vi "finalise_image.vi"(8 "error in (no error)":errorcluster, 9 "end of sweep?":bool, 11 "ImageAssemblerMG090623Binning in":refnum<class "ImageAssemblerMG090623Binning.lvclass">) -> (0 "error out":errorcluster, 3 "ImageAssemblerMG090623Binning out":refnum<class "ImageAssemblerMG090623Binning.lvclass">)   [LabVIEW 2010, in "ImageAssemblerMG090623Binning.lvclass"]
doc: "Finalises the image and sends it to registered observers. If the sweep is finished, a sweep terminator (empty Image array) is additionally send to observers."
uses:
  ImageAssemblerMG090623Binning.lvclass
  ImageAssemblerMG090623Binning.lvclass/ImageAssemblerMG090623Binning.ctl
  common/classes/Image/Image/Image.lvclass
  ImagingMode/GenericImagingMode/GenericImagingMode/GenericImagingMode.lvclass
  common/classes/GenericComponent/GenericComponent/class_data.vi
  common/classes/GenericComponent/GenericComponent/GenericComponent.lvclass
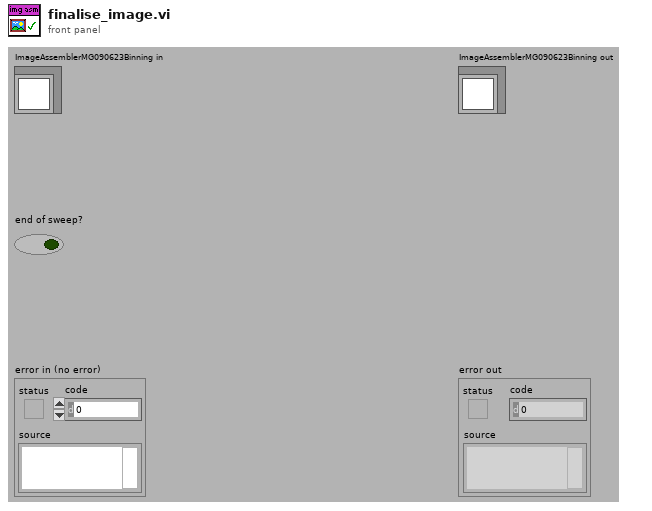
[diagram p1: front panel]
types:
  T1 = typedef "IMAQ Image.ctl" = refnum<image>
  T2 = typedef "GenericToplevelComponent.lvclass/common_trigger_enum.ctl" = enum16{"NULL", "initialise", "terminate", "fetch command", "fetch data", "attach observer", "register as observer", "detach observer", "acknowledge", "start", "stop", "sweep started", "sweep finished", "experiment started", "experiment stopped"}
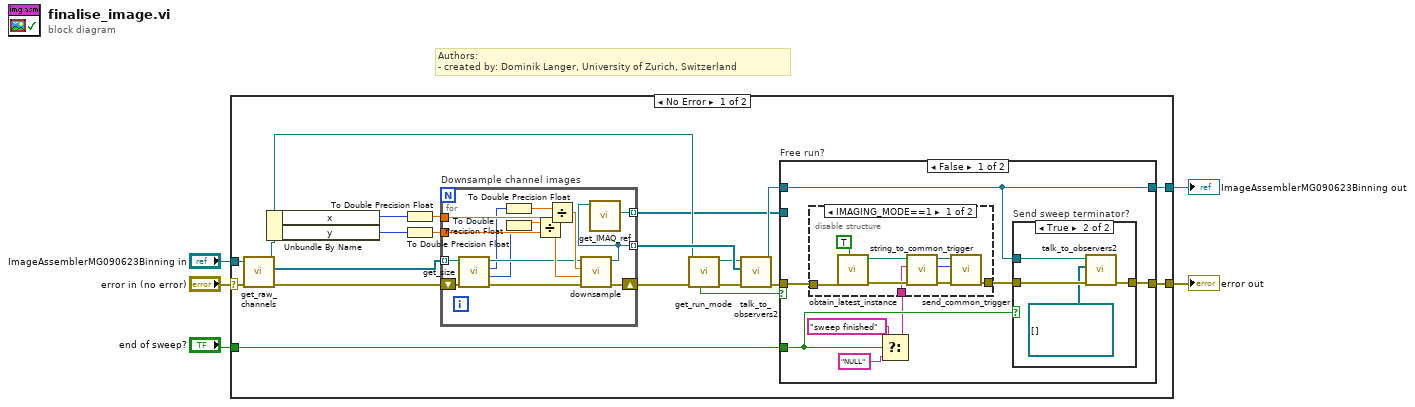
[diagram p0: block diagram]
diagram:
  # "Authors: \n- created by: Dominik Langer, University of Zurich, Switzerland"
  n1 = case shown="No Error" "error in (no error)" {
    selector: "error in (no error)" -> [w15 w67]
    tunnel: [w19 w67] -> w4
    tunnel: [w17 w66] -> w2
    tunnel: "ImageAssemblerMG090623Binning in" -> [w13 w66]
    tunnel: "end of sweep?" -> [w21 _]
    frame No Error {
      n2 = call-dynamic "get_raw_channels.vi"("error in (no error)"=w15, "DL090211ImageAssemblerScaffold.lvclass in"=w13) -> ("error out"=w14:errorcluster, "raw channels"=w11:refnum<class "Image.lvclass">[], "DL090211ImageAssemblerScaffold.lvclass out"=w12:refnum<class "ImageAssemblerMG090623Binning.lvclass">)  [unwired: 7 out]
      n3 = Unbundle By Name(w12) -> ("x"=w24:i32, "y"=w25:i32)
      n4 = To Double Precision Float(number=w24) -> (double precision float=w8:dbl)
      n5 = To Double Precision Float(number=w25) -> (double precision float=w7:dbl)
      n6 = for "Downsample channel images" {
        tunnel: w8 -> [w37]
        tunnel: w7 -> [w36]
        tunnel: w11 -> [w34] mode=indexing
        shift-right: [w28] -> w23
        shift-left: w14 -> [w35]
        tunnel: [w27] -> w16 mode=indexing
        tunnel: [w26] -> w6 mode=indexing
        n7 = call-dynamic "get_size.vi"("error in (no error)"=w35, "Image in"=w34) -> ("error out"=w40:errorcluster, "y resolution"=w31:i32, "x resolution"=w32:i32, "Image out"=w33:refnum<class "Image.lvclass">)  [unwired: 6 out]
        n8 = To Double Precision Float(number=w32) -> (double precision float=w29:dbl)
        n9 = To Double Precision Float(number=w31) -> (double precision float=w30:dbl)
        n10 = Divide(x=w30, y=w36) -> (x/y=w38:dbl)
        n11 = Divide(x=w29, y=w37) -> (x/y=w39:dbl)
        n12 = call-dynamic "downsample.vi"("error in (no error)"=w40, "y factor"=w38, "x factor"=w39, "Image in"=w33) -> ("error out"=w28:errorcluster, "Image out"=w27:refnum<class "Image.lvclass">)  [unwired: 6 out]
        n13 = call-dynamic "get_IMAQ_ref.vi"("Image.lvclass in"=w27) -> ("Image"=w26:T1)  [unwired: 6 in, 4 out]
      }
      n14 = call "get_run_mode.vi"("error in (no error)"=w23, "GenericPlugin in"=w12) -> ("error out"=w10:errorcluster, "GenericPlugin out"=w9:refnum<class "ImageAssemblerMG090623Binning.lvclass">, "is free run?"=w22:bool)  [unwired: 5 in, 2 out]
      n15 = call-dynamic "talk_to_observers2.vi"("error in (no error)"=w10, "image (channels)"=w16, "GenericToplevelComponent in"=w9) -> ("error out"=w20:errorcluster, "GenericToplevelComponent out"=w18:refnum<class "ImageAssemblerMG090623Binning.lvclass">)  [unwired: 7 in]
      n16 = case "Free run?" shown="False" w22 {
        tunnel: w20 -> [w48 w65]
        tunnel: [w46 w65] -> w19
        tunnel: w21 -> [w44 _]
        tunnel: w18 -> [w45 w64]
        tunnel: [w45 w64] -> w17
        tunnel: w6 -> [_ _]
        frame False {
          n17 = Select(t="sweep finished" ("message"), s=w44, f="NULL" ("message")) -> (s? t:f=w43:string)
          n18 = disable-structure shown="IMAGING_MODE==1" {
            disable-tunnel: w48 -> [w61 w63]
            disable-tunnel: [w60 w63] -> w47
            disable-tunnel: w43 -> [w54 _]
            frame condition #0 (active) {
              n19 = call "obtain_latest_instance.vi"("quick, but maybe outdated?"=TRUE, "error in (no error)"=w61) -> ("error out"=w59:errorcluster, "GenericScanMode out"=w57:refnum<class "GenericImagingMode.lvclass">)  [unwired: 8 in]
              n20 = call-dynamic "string_to_common_trigger.vi"("error in (no error)"=w59, "trigger string"=w54, "GenericToplevelComponent in"=w57) -> ("error out"=w58:errorcluster, "trigger"=w55:T2, "GenericToplevelComponent out"=w56:refnum<class "GenericImagingMode.lvclass">)  [unwired: 6 in]
              n21 = call-dynamic "send_common_trigger.vi"("error in (no error)"=w58, "trigger"=w55, "GenericToplevelComponent in"=w56) -> ("error out"=w60:errorcluster)  [unwired: 6 in, 2 out]
            }
            frame condition #1 {
            }
          }
          n22 = case "Send sweep terminator?" shown="True" w44 {
            tunnel: w47 -> [w49 w53]
            tunnel: [w49 w52] -> w46
            tunnel: w45 -> [_ w51]
            frame False {
            }
            frame True {
              n23 = call-dynamic "talk_to_observers2.vi"("error in (no error)"=w53, "image (channels)"=refnum<class "Image.lvclass">[] [], "GenericToplevelComponent in"=w51) -> ("error out"=w52:errorcluster)  [unwired: 7 in, 1 out]
            }
          }
        }
        frame True {
        }
      }
    }
    frame Error {
    }
  }
  "error out" <- w4
  "ImageAssemblerMG090623Binning out" <- w2
